vi "Sleep Stats.vi"(11 "Sleep Timers":u64[](array[numeric])) -> (3 "Stats":T1)   [LabVIEW 2021]
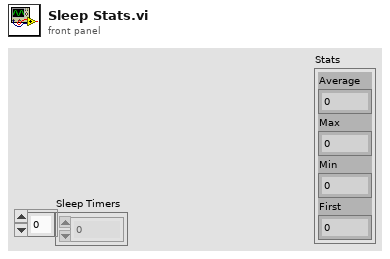
[diagram p1: front panel]
types:
  T1 = cluster{"Average":dbl, "Max":dbl, "Min":dbl, "First":dbl}
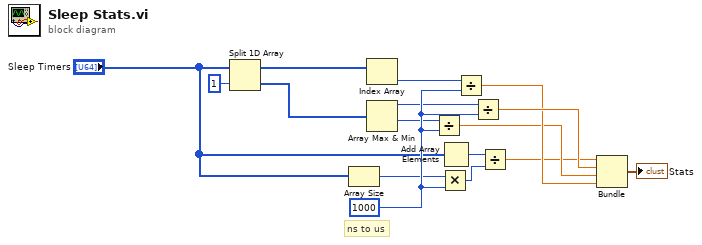
[diagram p0: block diagram]
diagram:
  w16 = u64 1000 ("y")
  # "ns to us"
  n1 = Split 1D Array(array="Sleep Timers", index=1) -> (first subarray=w5:u64[], second subarray=w6:u64[])
  n2 = Array Size(array="Sleep Timers") -> (size(s)=w2:i32)
  n3 = Index Array(array=w5) -> (element=w11:u64)  [unwired: 1 in]
  n4 = Array Max & Min(array=w6) -> (max value=w13:u64, min value=w9:u64)  [unwired: 2 out]
  n5 = Divide(x=w9, y=w16) -> (x/y=w10:dbl)
  n6 = Multiply(x=w2, y=w16) -> (x*y=w15:u64)
  n7 = Add Array Elements(numeric array="Sleep Timers") -> (sum=w7:u64)
  n8 = Divide(x=w11, y=w16) -> (x/y=w12:dbl)
  n9 = Divide(x=w13, y=w16) -> (x/y=w14:dbl)
  n10 = Divide(x=w7, y=w15) -> (x/y=w8:dbl)
  n11 = Bundle(w8, w14, w10, w12) -> (→"Stats":cluster{dbl, dbl, dbl, dbl})  [unwired: 1 in]
